vi "Calibration Cal Execute RF Test Fetch Results.vi"(8 "error in (no error)":errorcluster, 11 "Template Tx Test in":refnum<class "niDTS Calibration Cal Execute RF Test.lvclass">) -> (0 "error out":errorcluster, 2 "Results":T1, 3 "Template Tx Test out":refnum<class "niDTS Calibration Cal Execute RF Test.lvclass">)   [LabVIEW 2015, in "niDTS Utilities.lvlib" / "niDTS Calibration Cal Execute RF Test.lvclass"]
uses:
  niDTS Calibration Cal Execute RF Test.lvclass
  Includes/niDTS Calibration Cal Execute RF Test INC Results.ctl
  niDTS Calibration Cal Execute RF Test.lvclass/niDTS Calibration Cal Execute RF Test.ctl
  Calibration Cal Execute Get Cal Executed.vi
  niDTS Utilities.lvlib
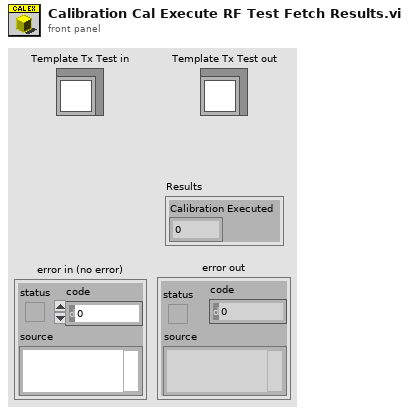
[diagram p1: front panel]
types:
  T1 = typedef "niDTS Utilities.lvlib/niDTS Calibration Cal Execute RF Test INC Results.ctl" = cluster{"Calibration Executed":u8}
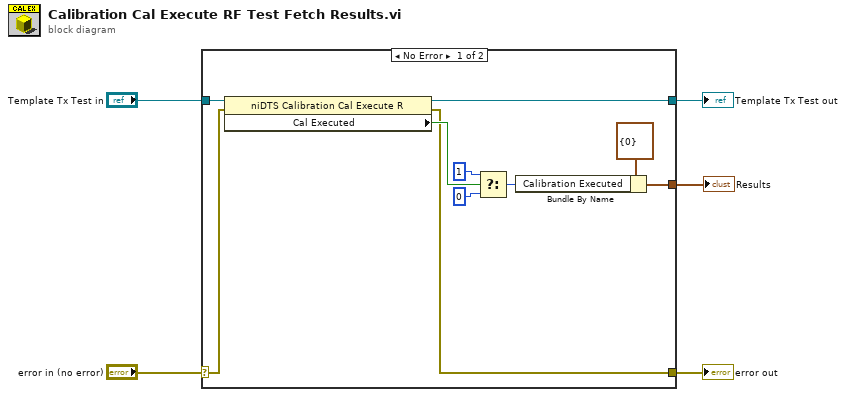
[diagram p0: block diagram]
diagram:
  n1 = case shown="No Error" "error in (no error)" {
    selector: "error in (no error)" -> [w7 w17]
    tunnel: [w6 w17] -> w4
    tunnel: [w12 w16] -> w2
    tunnel: "Template Tx Test in" -> [w13 w16]
    tunnel: [w14 _] -> w1
    frame No Error {
      n2 = property class="niDTS Calibration Cal Execute R"(reference=w13, error in=w7) -> (reference out=w12:refnum<class "niDTS Calibration Cal Execute RF Test.lvclass">, error out=w6:errorcluster, "Cal Executed"=w8:bool)
      n3 = Select(t=u8 1 ("Calibration Executed"), s=w8, f=u8 0 ("Calibration Executed")) -> (s? t:f=w9:u8)
      n4 = Bundle By Name(cluster=T1 {"Calibration Executed"=0} ("Results"), "Calibration Executed"=w9) -> (w14:T1)
    }
    frame Error {
    }
  }
  "error out" <- w4
  "Template Tx Test out" <- w2
  "Results" <- w1
